vi "unused_getType.vi"(8 "error in (no error)":errorcluster, 11 "Node In":refnum<class "Node.lvclass">) -> (0 "error out":errorcluster, 2 "type":refnum<vi>, 3 "Node Out":refnum<class "Node.lvclass">)   [LabVIEW 2023]
uses:
  Node.lvclass/Node.ctl
  Node.lvclass
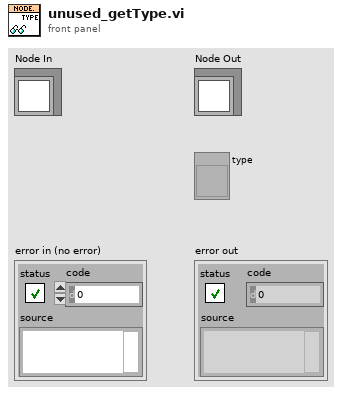
[diagram p1: front panel]
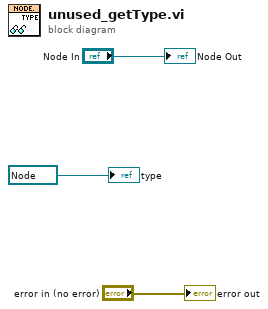
[diagram p0: block diagram]
diagram:
  "error out" <- "error in (no error)"
  "Node Out" <- "Node In"
  "type" <- refnum<vi> refnum ("type")
